vi "Set Project Version.vi"(0 "Major":i32=2, 5 "Minor":string, 7 "Fix":i32) -> (4 "semver":string, 8 "build specs":refnum<vi>[](array[refnum]), 15 "error out":errorcluster)   [LabVIEW 2020]
uses:
  <vilib>/regexp/Match Regular Expression.xnode
panel:
  out "Path":path
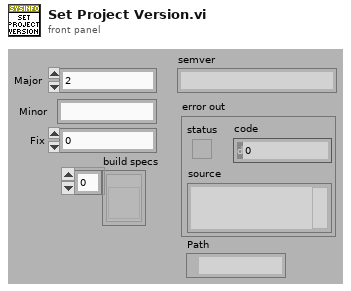
[diagram p1: front panel]
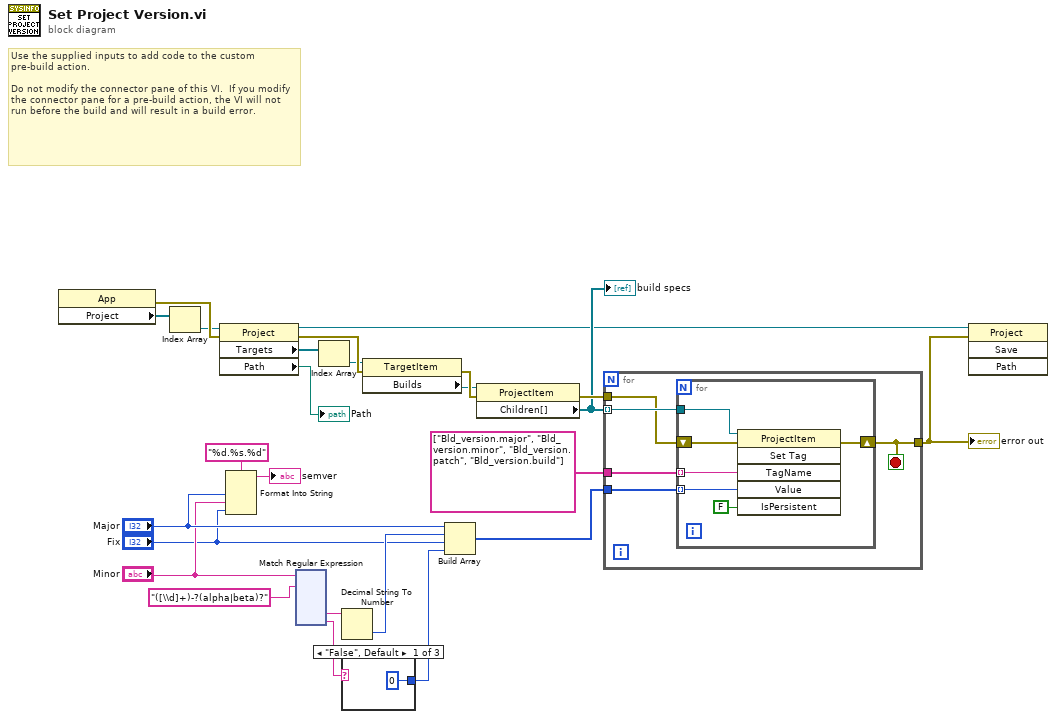
[diagram p0: block diagram]
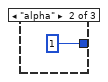
[diagram p2: hidden frame]
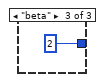
[diagram p3: hidden frame]
diagram:
  # "Use the supplied inputs to add code to the custom pre-build action.\n\nDo not modify the connector pane of this VI.  If you modify the connector pane for a pre-build action, the VI will not run before the build and will result in a build error."
  n1 = property class="App"() -> (error out=w25:errorcluster, "Project"=w22:refnum<vi>[])  [unwired: 2 in, 1 out]
  n2 = Index Array(array=w22) -> (element=w21:refnum<vi>)  [unwired: 1 in]
  n3 = property class="Project"(reference=w21, error in=w25) -> (reference out=w14:refnum<vi>, error out=w24:errorcluster, "Targets"=w20:refnum<vi>[], "Path"=→"Path":path)
  n4 = Format Into String(format string="%d.%s.%d", "Major", "Minor", "Fix") -> (resulting string=→"semver":string)  [unwired: 2 in, 1 out]
  n5 = xnode "Match Regular Expression"("input string"="Minor", "regular expression"="([\\d]+)-?(alpha|beta)?") -> ("submatch 1"=w10:string, "submatch 2"=w8:string)  [unwired: 4 in, 5 out]
  n6 = Index Array(array=w20) -> (element=w19:refnum<vi>)  [unwired: 1 in]
  n7 = Decimal String To Number(string=w10) -> (number=w9:i32)  [unwired: 2 in, 1 out]
  n8 = case shown="\"False\", Default" w8 {
    tunnel: [0 1 2] -> w7
    frame "False", Default {
    }
    frame "alpha" {
    }
    frame "beta" {
    }
  }
  n9 = property class="TargetItem"(reference=w19, error in=w24) -> (error out=w23:errorcluster, "Builds"=w18:refnum<vi>)  [unwired: 1 out]
  n10 = Build Array("Major", w9, "Fix", w7) -> (w12:i32[])
  n11 = property class="ProjectItem"(reference=w18, error in=w23) -> (error out=w17:errorcluster, "Children[]"=w16:refnum<vi>[])  [unwired: 1 out]
  "build specs" <- w16
  n12 = for {
    tunnel: w17 -> [w32]
    tunnel: w16 -> [w33] mode=indexing
    tunnel: [w31] -> w15
    tunnel: w12 -> [w30]
    tunnel: string[] ["Bld_version.major", "Bld_version.minor", "Bld_version.patch", "Bld_version.build"] -> [w29]
    stop <- w31 stop-if-true
    n13 = for {
      tunnel: w33 -> [w38]
      tunnel: w30 -> [w35] mode=indexing
      shift-right: [w36] -> w31
      shift-left: w32 -> [w37]
      tunnel: w29 -> [w34] mode=indexing
      n14 = invoke class="ProjectItem" method="Set Tag"(reference=w38, error in=w37, "TagName"=w34, "Value"=w35, "IsPersistent"=FALSE ("Is Persistent")) -> (error out=w36:errorcluster)  [unwired: 1 in, 5 out]
    }
  }
  "error out" <- w15
  n15 = invoke class="Project" method="Save"(reference=w14, error in=w15) -> ()  [unwired: 2 in, 4 out]
